vi "test_PXI simple test.vi"() -> ()   [LabVIEW 2023]
uses:
  Measure and Stimulus Subsystems/Measure and Stimulus Subsystems.lvclass
  <vilib>/Waveform/WDTOps.llb/WDT Number of Waveform Samples DBL.vi
panel:
  out "total samples fetched":i32
  out "#samples fetched":i32[](array[numeric])
  out "Iteration":i32
  in  "Stop":bool
  out "Photosensor Waveform Chart":waveform(dbl)(graph)
  out "Error Out":errorcluster
  out "Powersensor Scalar":dbl
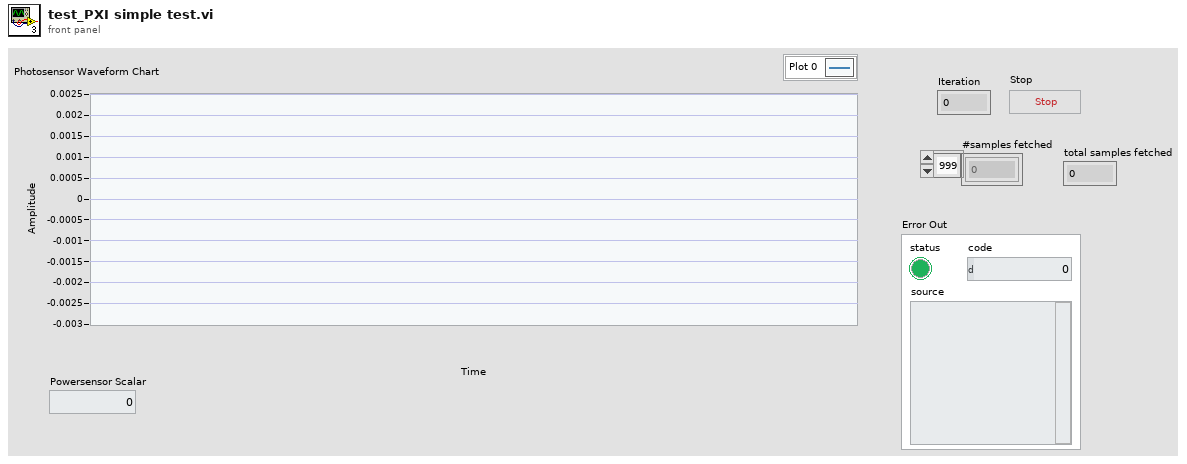
[diagram p1: front panel]
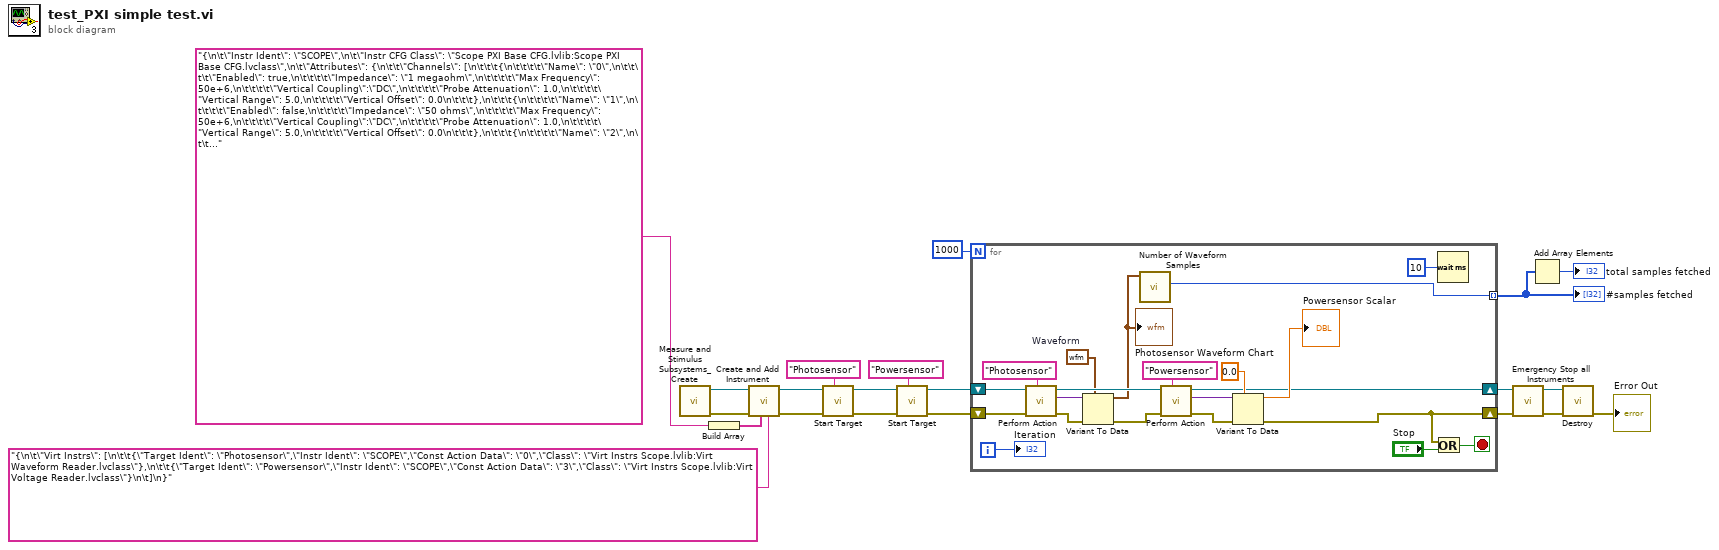
[diagram p0: block diagram]
diagram:
  n1 = call "Measure and Stimulus Subsystems_Create.vi"() -> ("Error Out"=w20:errorcluster, "reference out"=w21:refnum<class "Measure and Stimulus Subsystems.lvclass">)  [unwired: 10 in]
  n2 = Build Array("{\n\t\"Instr Ident\": \"SCOPE\",\n\t\"Instr CFG Class\": \"Scope PXI Base CFG.lvlib:Scope PXI Base CFG.lvclass\",\n\t\"Attributes\": {\n\t\t\"Channels\": [\n\t\t\t{\n\t\t\t\t\"Name\": \"0\",\n\t\t\t\t\"Enabled\": true,\n\t\t\t\t\"Impedance\": \"1 megaohm\",\n\t\t\t\t\"Max Frequency\": 50e+6,\n\t\t\t\t\"Vertical Coupling\":\"DC\",\n\t\t\t\t\"Probe Attenuation\": 1.0,\n\t\t\t\t\"Vertical Range\": 5.0,\n\t\t\t\t\"Vertical Offset\": 0.0\n\t\t\t},\n\t\t\t{\n\t\t\t\t\"Name\": \"1\",\n\t\t\t\t\"Enabled\": false,\n\t\t\t\t\"Impedance\": \"50 ohms\",\n\t\t\t\t\"Max Frequency\": 50e+6,\n\t\t\t\t\"Vertical Coupling\":\"DC\",\n\t\t\t\t\"Probe Attenuation\": 1.0,\n\t\t\t\t\"Vertical Range\": 5.0,\n\t\t\t\t\"Vertical Offset\": 0.0\n\t\t\t},\n\t\t\t{\n\t\t\t\t\"Name\": \"2\",\n\t\t\t\t\"Enabled\": false,\n\t\t\t\t\"Impedance\": \"50 ohms\",\n\t\t\t\t\"Max Frequency\": 50e+6,\n\t\t\t\t\"Vertical Coupling\":\"DC\",\n\t\t\t\t\"Probe Attenuation\": 1.0,\n\t\t\t\t\"Vertical Range\": 5.0,\n\t\t\t\t\"Vertical Offset\": 0.0\n\t\t\t},\n\t\t\t{\n\t\t\t\t\"Name\": \"3\",\n\t\t\t\t\"Enabled\": true,\n\t\t\t\t\"Impedance\": \"50 ohms\",\n\t\t\t\t\"Max Frequency\": 50e+6,\n\t\t\t\t\"Vertical Coupling\":\"DC\",\n\t\t\t\t\"Probe Attenuation\": 1.0,\n\t\t\t\t\"Vertical Range\": 1.4,\n\t\t\t\t\"Vertical Offset\": 0.0\n\t\t\t},\n\t\t\t{\n\t\t\t\t\"Name\": \"4\",\n\t\t\t\t\"Enabled\": false,\n\t\t\t\t\"Impedance\": \"50 ohms\",\n\t\t\t\t\"Max Frequency\": 50e+6,\n\t\t\t\t\"Vertical Coupling\":\"DC\",\n\t\t\t\t\"Probe Attenuation\": 1.0,\n\t\t\t\t\"Vertical Range\": 5.0,\n\t\t\t\t\"Vertical Offset\": 0.0\n\t\t\t},\n\t\t\t{\n\t\t\t\t\"Name\": \"5\",\n\t\t\t\t\"Enabled\": false,\n\t\t\t\t\"Impedance\": \"50 ohms\",\n\t\t\t\t\"Max Frequency\": 50e+6,\n\t\t\t\t\"Vertical Coupling\":\"DC\",\n\t\t\t\t\"Probe Attenuation\": 1.0,\n\t\t\t\t\"Vertical Range\": 5.0,\n\t\t\t\t\"Vertical Offset\": 0.0\n\t\t\t},\n\t\t\t{\n\t\t\t\t\"Name\": \"6\",\n\t\t\t\t\"Enabled\": false,\n\t\t\t\t\"Impedance\": \"50 ohms\",\n\t\t\t\t\"Max Frequency\": 50e+6,\n\t\t\t\t\"Vertical Coupling\":\"DC\",\n\t\t\t\t\"Probe Attenuation\": 1.0,\n\t\t\t\t\"Vertical Range\": 5.0,\n\t\t\t\t\"Vertical Offset\": 0.0\n\t\t\t},\n\t\t\t{\n\t\t\t\t\"Name\": \"7\",\n\t\t\t\t\"Enabled\": false,\n\t\t\t\t\"Impedance\": \"50 ohms\",\n\t\t\t\t\"Max Frequency\": 50e+6,\n\t\t\t\t\"Vertical Coupling\":\"DC\",\n\t\t\t\t\"Probe Attenuation\": 1.0,\n\t\t\t\t\"Vertical Range\": 5.0,\n\t\t\t\t\"Vertical Offset\": 0.0\n\t\t\t}\n\t\t],\n\t\t\"Horizontal\": {\n\t\t\t\"Enforce Realtime\": true,\n\t\t\t\"Number of Records\": 1,\n\t\t\t\"Min Sample Rate\": 1e+5,\n\t\t\t\"Reference Position\":10, //percent\n\t\t\t\"Min Record Length\":1e+3\n\t\t},\n\t\t\"Acquire\": {\n\t\t\t\"Type\": \"Normal\",\n\t\t\t\"NumSamples\": 1e+4,\n  \t\"Fetch Relative To\": \"Read Pointer\" \n\t\t},\n\t\t\"Export Signal\": {\n\t\t\t\"Signal Identifier\": \"None\",\n\t\t\t\"Signal\": \"None\",\n\t\t\t\"Output Terminal\": \"None\"\n\t\t},\n\t\t\"Trigger\": {\n\t\t\t\"Type\": \"Software\",\n\t\t\t\"Slope\": \"Positive\",\n\t\t\t\"Source\": \"RTSI 0\",\n\t\t\t\"Holdoff\": 0.0,\n\t\t\t\"Delay\": 0.0\n\t\t}\n\t}\n}") -> (w7:string[])
  n3 = call "Create and Add Instrument.vi"(4:"{\n\t\"Virt Instrs\": [\n\t\t{\"Target Ident\": \"Photosensor\",\"Instr Ident\": \"SCOPE\",\"Const Action Data\": \"0\",\"Class\": \"Virt Instrs Scope.lvlib:Virt Waveform Reader.lvclass\"},\n\t\t{\"Target Ident\": \"Powersensor\",\"Instr Ident\": \"SCOPE\",\"Const Action Data\": \"3\",\"Class\": \"Virt Instrs Scope.lvlib:Virt Voltage Reader.lvclass\"}\n\t]\n}", "Physical Intr Configs"=w7, "Error In"=w20, "reference in"=w21) -> ("Error Out"=w19:errorcluster, "reference out"=w10:refnum<class "Measure and Stimulus Subsystems.lvclass">)  [unwired: 6 in]
  n4 = call "Start Target.vi"("Target Ident"="Photosensor" ("Target Identifier"), "Error In"=w19, "reference in"=w10) -> ("Error Out"=w11:errorcluster, "reference out"=w3:refnum<class "Measure and Stimulus Subsystems.lvclass">)  [unwired: 7 in]
  n5 = call "Start Target.vi"("Target Ident"="Powersensor", "Error In"=w11, "reference in"=w3) -> ("Error Out"=w4:errorcluster, "reference out"=w2:refnum<class "Measure and Stimulus Subsystems.lvclass">)  [unwired: 7 in]
  n6 = for {
    N: 1000 -> [_]
    shift-right: [w27] -> w14
    shift-left: w4 -> [w37]
    shift-right: [w25] -> w17
    shift-left: w2 -> [w36]
    tunnel: [w22] -> w6 mode=indexing
    i -> [w24]
    stop <- w26 stop-if-true
    w33 = waveform(dbl) {"t0"=timestamp(0 s since 1904-01-01), "dt"=1.0, "Y"=[]}  # Waveform
    n7 = call "Perform Action.vi"("Target Ident"="Photosensor" ("Target Identifier"), "Error In"=w37, "reference in"=w36) -> ("Error Out"=w40:errorcluster, "Output"=w34:variant, "reference out"=w41:refnum<class "Measure and Stimulus Subsystems.lvclass">)  [unwired: 6 in]
    n8 = Variant To Data(error in=w40, type=w33, Variant=w34) -> (data=w23:waveform(dbl), error out=w35:errorcluster)
    "Photosensor Waveform Chart" <- w23
    n9 = call-poly <vilib>:"Number of Waveform Samples.vi"("waveform in"=w23) -> ("number of samples"=w22:i32)  [unwired: 8 in, 2 out]
    n10 = call "Perform Action.vi"("Target Ident"="Powersensor" ("Target Identifier"), "Error In"=w35, "reference in"=w41) -> ("Error Out"=w38:errorcluster, "Output"=w32:variant, "reference out"=w25:refnum<class "Measure and Stimulus Subsystems.lvclass">)  [unwired: 6 in]
    n11 = Variant To Data(error in=w38, type=0.0, Variant=w32) -> (data=→"Powersensor Scalar":dbl, error out=w27:errorcluster)
    n12 = Or(x=w27, y="Stop") -> (x .or. y?=w26:bool)
    n13 = Wait (ms)(milliseconds to wait=u32 10) -> ()  [unwired: 1 out]
    "Iteration" <- w24
  }
  "#samples fetched" <- w6
  n14 = call "Emergency Stop all Instruments.vi"("Error In"=w14, "reference in"=w17) -> ("Error Out"=w18:errorcluster, "reference out"=w16:refnum<class "Measure and Stimulus Subsystems.lvclass">)  [unwired: 8 in]
  n15 = Add Array Elements(numeric array=w6) -> (sum=→"total samples fetched":i32)
  n16 = call "Destroy.vi"("Error In"=w18, "reference in"=w16) -> ("Error Out"=→"Error Out":errorcluster)  [unwired: 8 in, 1 out]
